vi "Set Coefficient Caps.vi"(0 "Session Handle":T1, 5 "Ki Error":u16, 7 "Kd Error":u16, 9 "Max Cap":u16, 11 "error in (no error)":errorcluster) -> (4 "Session Handle Out":T1, 15 "error out":errorcluster)   [LabVIEW 2015, in "Peltier.lvclass"]
uses:
  Peltier.lvclass
  Typedefs/Session Handle.ctl
  PAS/PAS.lvclass
panel:
  out "Success?":bool
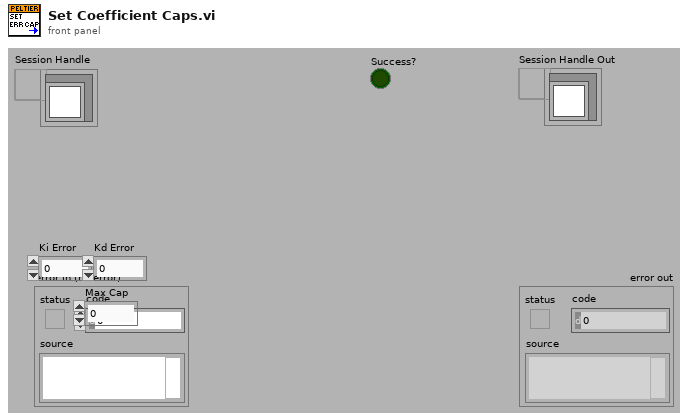
[diagram p1: front panel]
types:
  T1 = typedef "Peltier.lvclass/Session Handle.ctl" = refnum<data-value>
  T2 = typedef "XNET Frame CAN.ctl" = cluster{"timestamp":timestamp, "payload":u8[], "identifier":u32, "type":T3, "extended?":bool, "echo?":bool}
  T3 = typedef "XNET Frame Type CAN.ctl" = u8
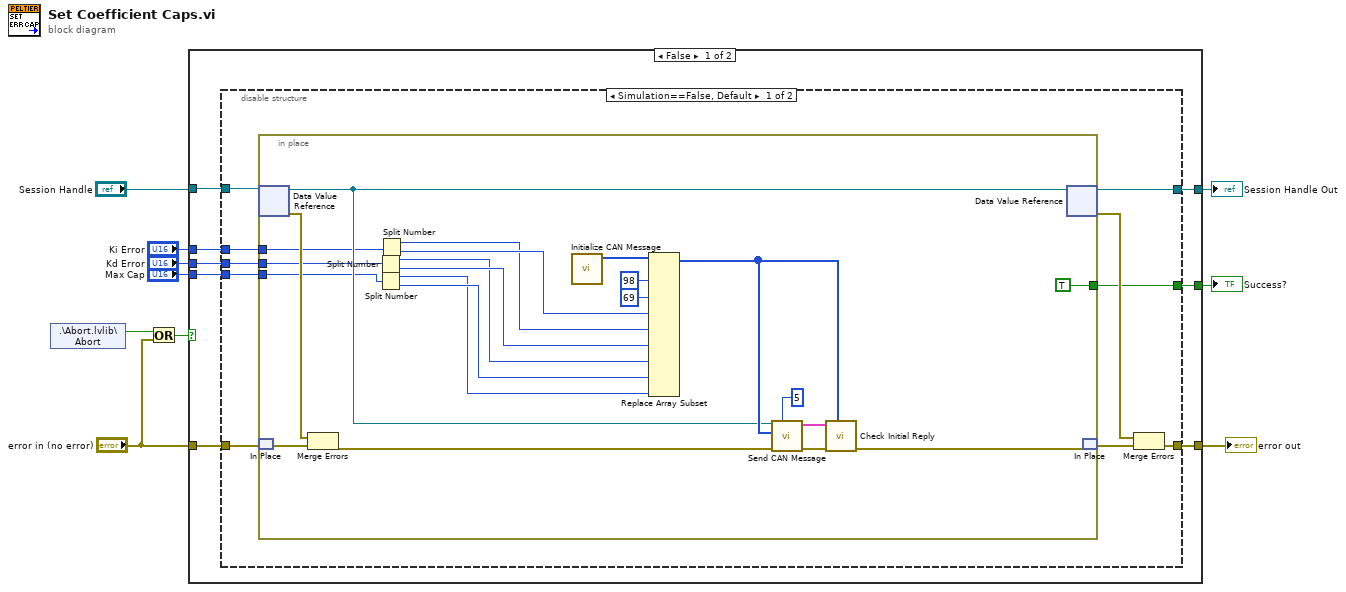
[diagram p0: block diagram]
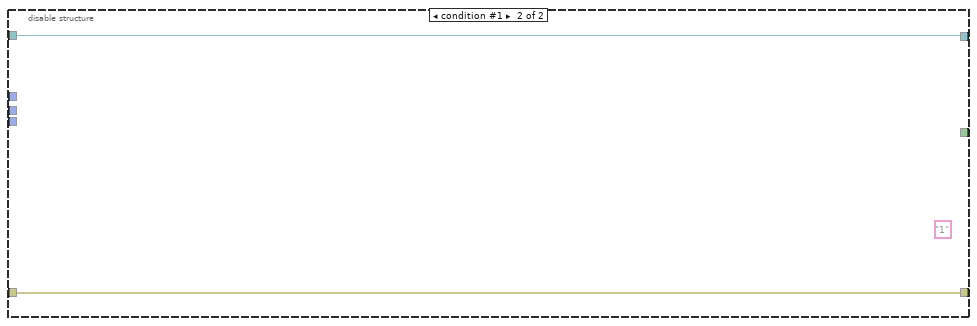
[diagram p2: hidden frame]
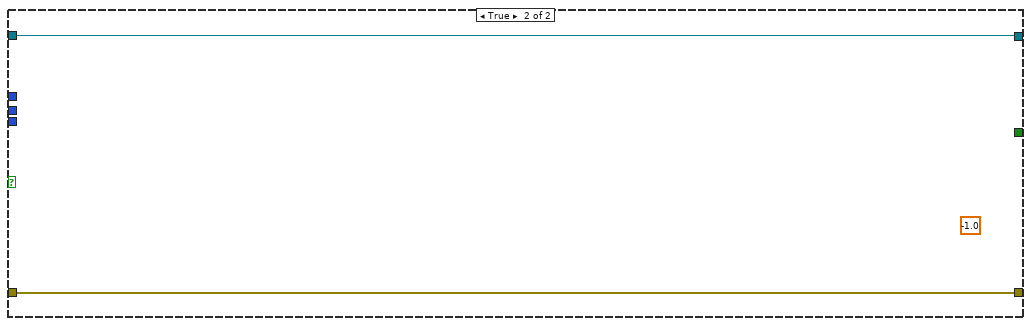
[diagram p3: hidden frame]
diagram:
  n1 = shared-variable ".\\Abort.lvlib\\Abort"() -> (w9:bool)  [unwired: 1 in, 1 out]
  n2 = Or(x=w9, y="error in (no error)") -> (x .or. y?=w7:bool)
  n3 = case shown="False" w7 {
    tunnel: [w18 w54] -> w5
    tunnel: [w17 w53] -> w10
    tunnel: "Session Handle" -> [w16 w54]
    tunnel: "error in (no error)" -> [w15 w53]
    tunnel: [w14 _] -> w4
    tunnel: "Ki Error" -> [w13 _]
    tunnel: "Kd Error" -> [w12 _]
    tunnel: "Max Cap" -> [w11 _]
    frame False {
      n4 = disable-structure shown="Simulation==False, Default" {
        disable-tunnel: [w28 w52] -> w18
        disable-tunnel: [w25 w51] -> w17
        disable-tunnel: w16 -> [w24 w52]
        disable-tunnel: w15 -> [w23 w51]
        disable-tunnel: [w22 _] -> w14
        disable-tunnel: w13 -> [w21 _]
        disable-tunnel: w12 -> [w20 _]
        disable-tunnel: w11 -> [w19 _]
        frame condition #0 (active) {
          n5 = in-place {
            in-place-border: [TRUE] -> w22
            in-place-border: w21 -> [w39]
            in-place-border: w20 -> [w36]
            in-place-border: w19 -> [w33]
            n6 = in-place-dvr #1(w24) -> (w43:refnum<class "Peltier.lvclass">, w48:errorcluster)
            n7 = in-place-match #2(w23) -> (w47:errorcluster)
            n8 = Merge Errors(w48, w47) -> (w42:errorcluster)
            n9 = Split Number(x=w36) -> (hi(x)=w34:u8, lo(x)=w35:u8)
            n10 = Split Number(x=w33) -> (hi(x)=w31:u8, lo(x)=w32:u8)
            n11 = Split Number(x=w39) -> (hi(x)=w37:u8, lo(x)=w38:u8)
            n12 = call "Initialize CAN Message.vi"() -> ("Initial Payload"=w49:u8[])  [unwired: 11 in]
            n13 = Replace Array Subset(array=w49, new element #1=u8 98 ("new element/subarray"), new element #2=u8 69 ("new element/subarray"), new element #3=w38, new element #4=w37, new element #5=w35, new element #6=w34, new element #7=w32, new element #8=w31) -> (w46:u8[])  [unwired: 8 in]
            n14 = call "Send CAN Message.vi"("Number of Retries"=5, "error in (no error)"=w42, "payload"=w46, "Peltier In"=w43) -> ("error out"=w30:errorcluster, "Reply"=w44:T2[])  [unwired: 5 in, 1 out]
            n15 = call "Check Initial Reply.vi"("Write Message"=w46, "error in (no error)"=w30, "Reply"=w44) -> ("error out"=w29:errorcluster)  [unwired: 5 in, 3 out]
            n16 = in-place-dvr #1(w43) -> (w28:T1, w26:errorcluster)
            n17 = in-place-match #2(w29) -> (w27:errorcluster)
          }
          n18 = Merge Errors(w26, w27) -> (w25:errorcluster)
        }
        frame condition #1 {
          (unwired) "1"
        }
      }
    }
    frame True {
      (unwired) -1.0
    }
  }
  "error out" <- w10
  "Success?" <- w4
  "Session Handle Out" <- w5
